vi "PFE Panel.vi"(8 "error in (no error)":errorcluster, 9 "PFE Configuration (\"\")":string, 10 "PFE Position In":variant, 11 "PFE Command":T1) -> (0 "error out":errorcluster, 1 "PFE Flat Output":string, 2 "PFE Position Out":variant)   [LabVIEW 2011]
uses:
  PFE Command.ctl
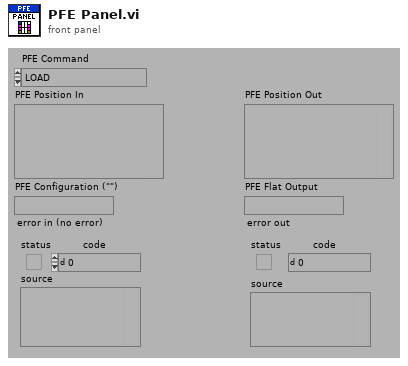
[diagram p1: front panel]
types:
  T1 = typedef "PFE Command.ctl" = enum16{"LOAD", "INITIALIZE", "PRESET", "SET STIMULUS", "GET STIMULUS", "GET INFO", "RELEASE", "UNLOAD"}
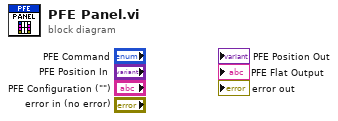
[diagram p0: block diagram]
diagram:
